vi "LabVIEW_hiss_1.vi"() -> ()   [LabVIEW 2020]
uses:
  States_1.ctl
panel:
  in  "Meta nödstopp":bool
  in  "?":bool
  in  "Tab Control":enum32{"Hisspanel", "Inställningar"}(tab)
  in  "Våningar":T1
  out "Nuvarande Våning":T2
  out "Våningshöjd":dbl
  out "Våningstolerans":dbl
  in  "Potentiometervärden":T3={"Högsta våning"=10.0, "Lägsta våning"=0.0}
  in  "GPIB-addresser":T4={"Funktionsgenerator"="1", "Multimeter"="3", "Nätaggregat"="2"}
  in  "Antal våningar":i32=5
  in  "Tolerans Rel. Våningshöjd":i32=5
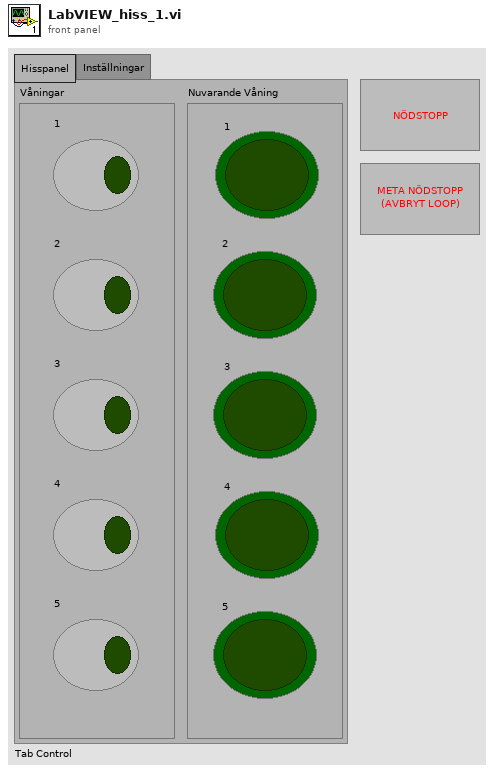
[diagram p1: front panel]
types:
  T1 = cluster{"1":bool, "2":bool, "3":bool, "4":bool, "5":bool}
  T2 = cluster{"1":bool, "\n2":bool, "3":bool, "4":bool, "5":bool}
  T3 = cluster{"Högsta våning":dbl, "Lägsta våning":dbl}
  T4 = cluster{"Funktionsgenerator":string, "Multimeter":string, "Nätaggregat":string}
  T5 = cluster{"Våningshöjd":dbl, "Våningstolerans":dbl, "Högsta våning":dbl, "Lägsta våning":dbl}
  T6 = typedef "States_1.ctl" = enum16{"Initialtillstånd", "Kör ner", "Kör upp", "Vänta på input", "Spela ljudfil", "Nödstopp"}
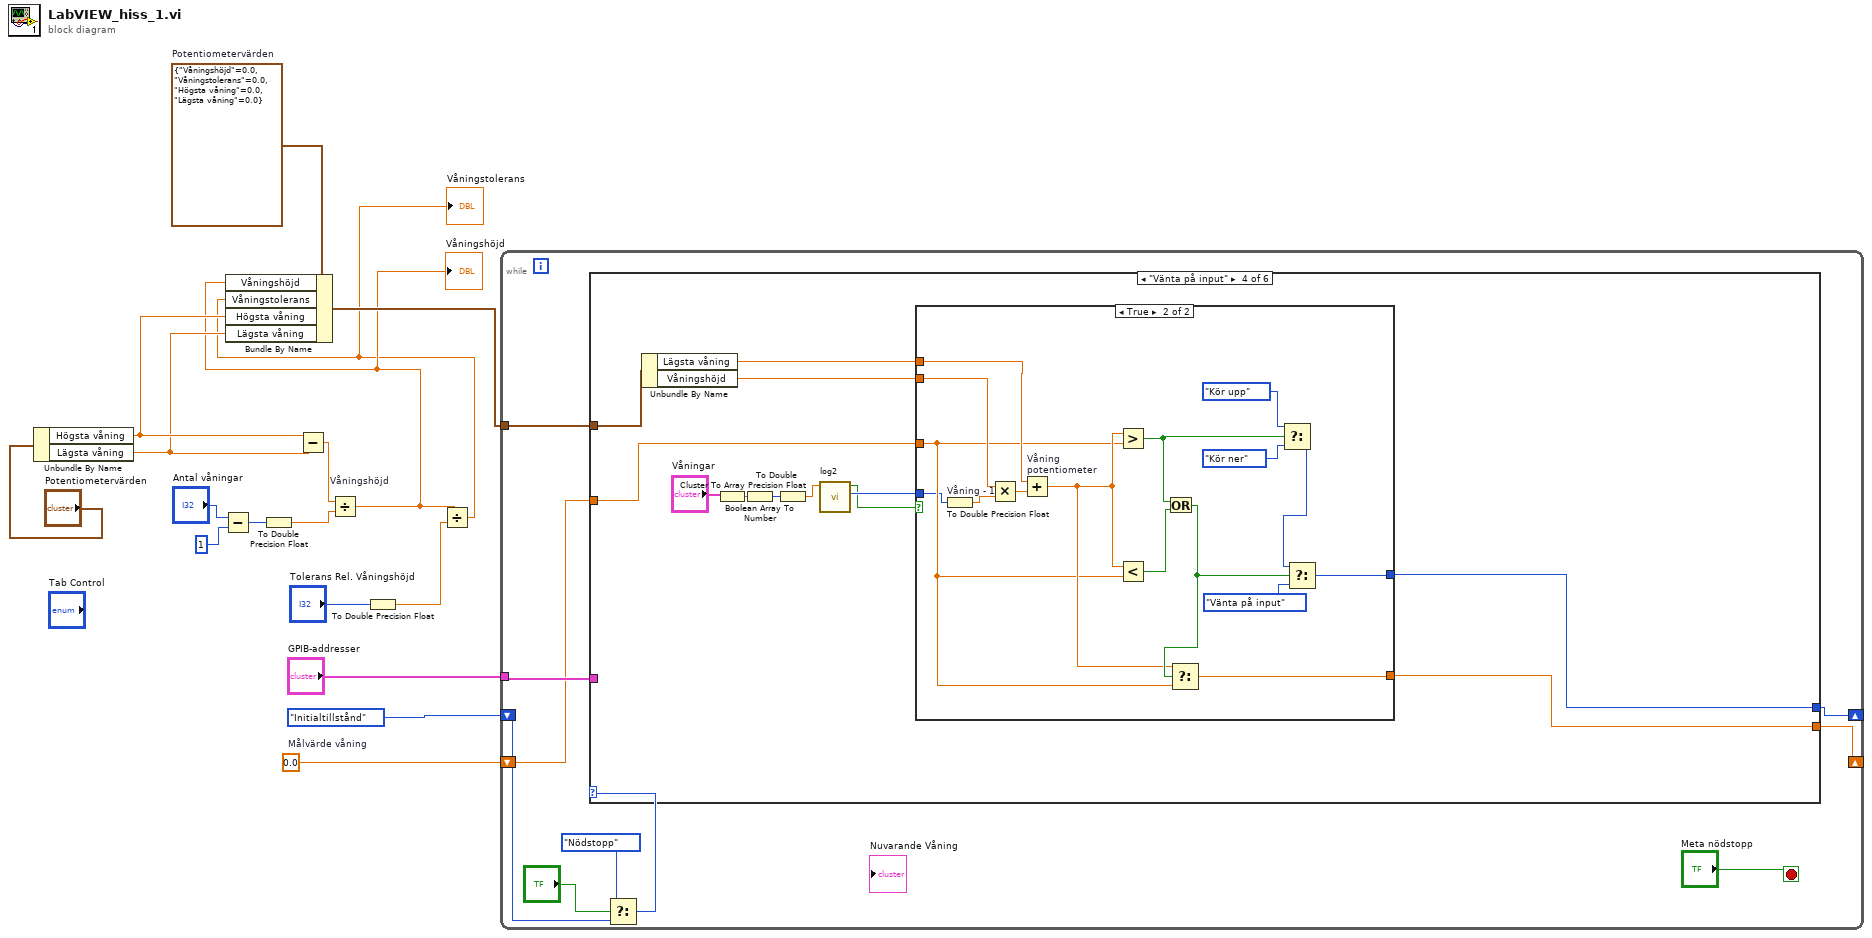
[diagram p0: block diagram]
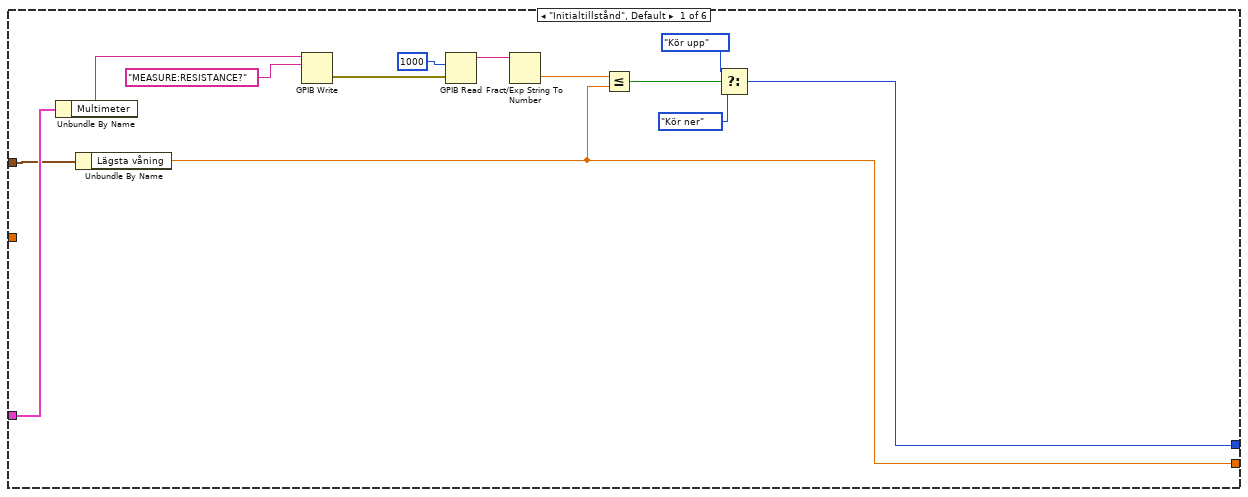
[diagram p2: hidden frame]
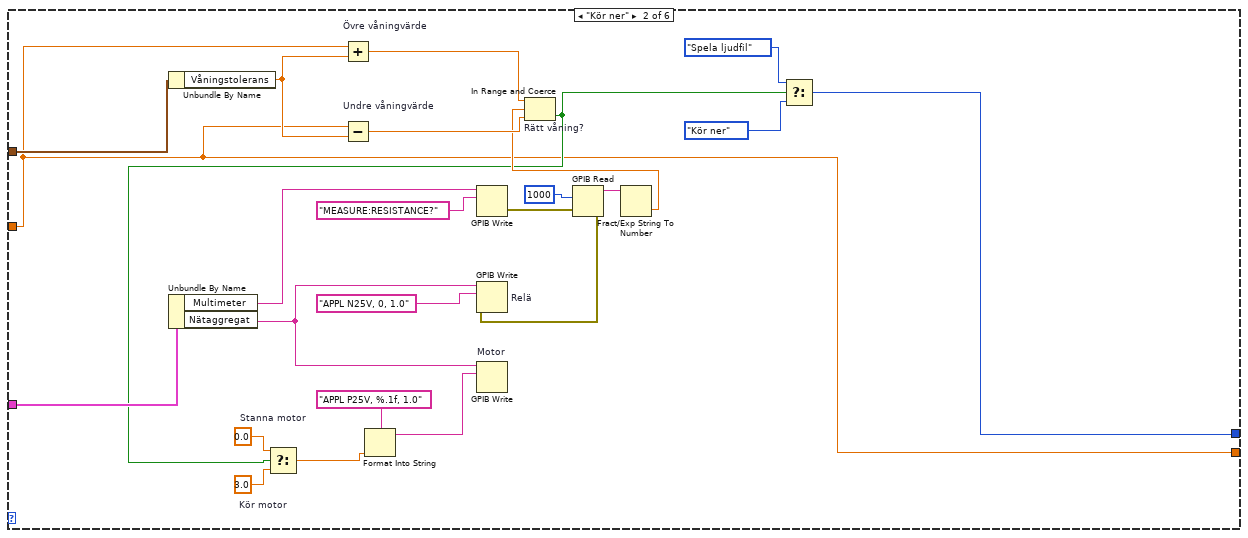
[diagram p3: hidden frame]
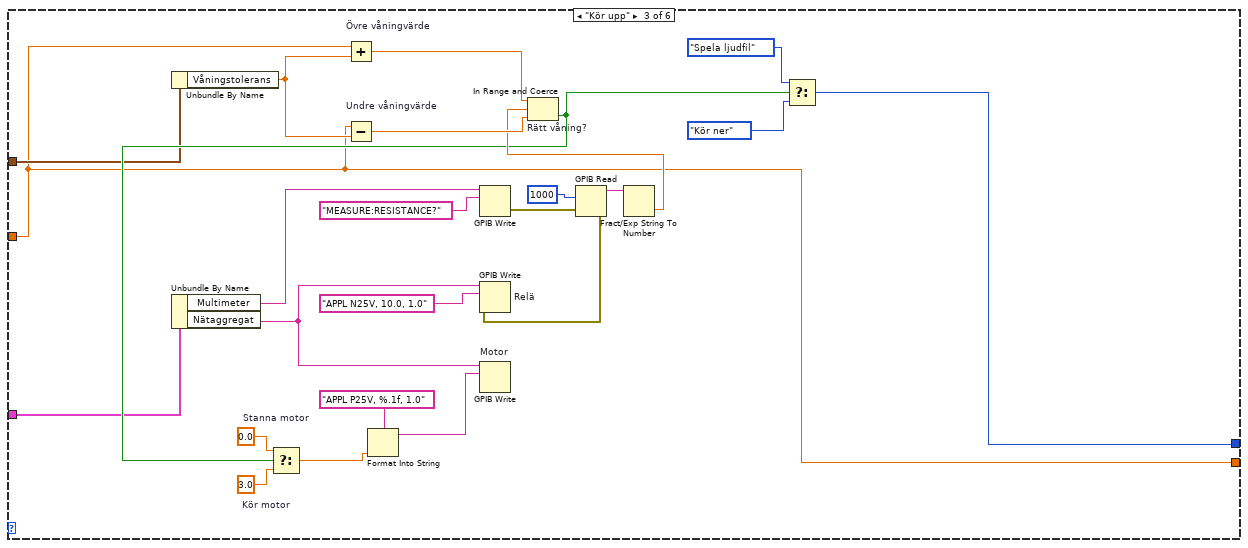
[diagram p4: hidden frame]
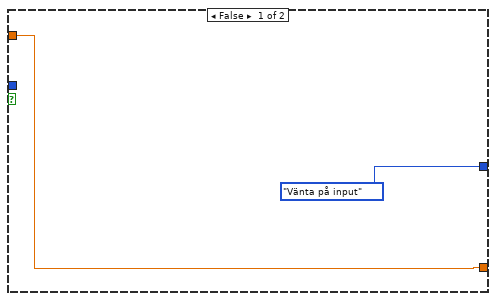
[diagram p5: hidden frame]
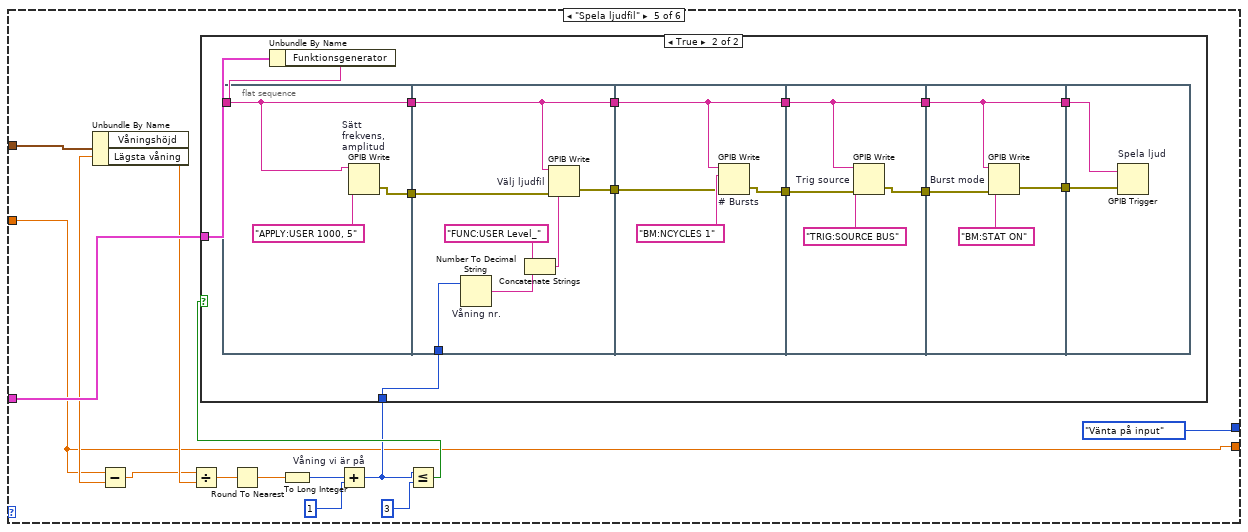
[diagram p6: hidden frame]
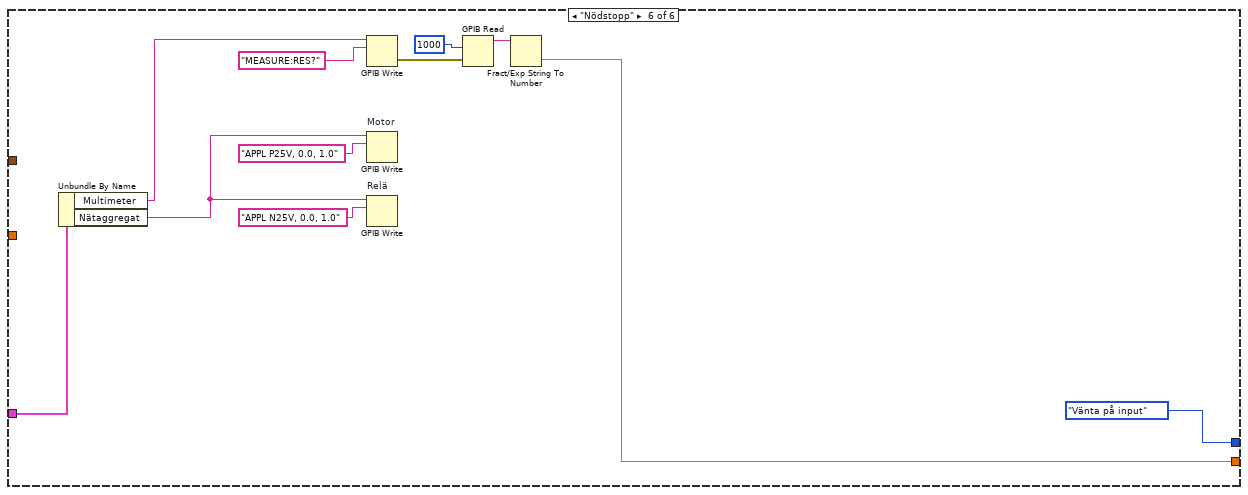
[diagram p8: hidden frame]
diagram:
  w16 = 0.0  # Målvärde våning
  w10 = T5 {"Våningshöjd"=0.0, "Våningstolerans"=0.0, "Högsta våning"=0.0, "Lägsta våning"=0.0}  # Potentiometervärden
  n1 = Unbundle By Name("Potentiometervärden") -> ("Högsta våning"=w5:dbl, "Lägsta våning"=w4:dbl)
  n2 = Subtract(x="Antal våningar", y=1) -> (x-y=w13:i32)
  n3 = To Double Precision Float(number=w13) -> (double precision float=w12:dbl)
  n4 = Subtract(x=w5, y=w4) -> (x-y=w14:dbl)
  n5 = Divide "Våningshöjd"(x=w14, y=w12) -> (x/y=w3:dbl)
  "Våningshöjd" <- w3
  n6 = To Double Precision Float(number="Tolerans Rel. Våningshöjd") -> (double precision float=w11:dbl)
  n7 = Divide(x=w3, y=w11) -> (x/y=w2:dbl)
  "Våningstolerans" <- w2
  n8 = Bundle By Name(cluster=w10, "Våningshöjd"=w3, "Våningstolerans"=w2, "Högsta våning"=w5, "Lägsta våning"=w4) -> (w9:T5)
  n9 = while {
    shift-right: [w22] -> _
    shift-left: States_1."Initialtillstånd" -> [w26]
    tunnel: "GPIB-addresser" -> [w23]
    shift-right: [w21] -> _
    shift-left: w16 -> [w19]
    tunnel: w9 -> [w20]
    stop <- "Meta nödstopp" stop-if-true
    n10 = Select(t=States_1."Nödstopp", s="?", f=w26) -> (s? t:f=w24:T6)
    n11 = case shown="\"Vänta på input\"" w24 {
      tunnel: w23 -> [w40 w63 w66 _ w130 w178]
      tunnel: [w30 w43 w65 w92 States_1."Vänta på input" States_1."Vänta på input"] -> w22
      tunnel: [w29 w41 w64 w90 w117 w170] -> w21
      tunnel: w20 -> [w28 w58 w67 w95 w129 _]
      tunnel: w19 -> [_ w41 w64 w91 w117 _]
      frame "Initialtillstånd", Default {
        n12 = Unbundle By Name(w40) -> ("Multimeter"=w39:string)
        n13 = Unbundle By Name(w28) -> ("Lägsta våning"=w29:dbl)
        n14 = GPIB Write(0:w39, 1:"MEASURE:RESISTANCE?") -> (6:w37:errorcluster)  [unwired: 3 in, 1 out]
        n15 = GPIB Read(1:1000, 3:w37) -> (5:w35:string)  [unwired: 3 in, 2 out]
        n16 = Fract/Exp String To Number(string=w35) -> (number=w34:dbl)  [unwired: 3 in, 1 out]
        n17 = Less Or Equal?(x=w34, y=w29) -> (x <= y?=w33:bool)
        n18 = Select(t=States_1."Kör upp", s=w33, f=States_1."Kör ner") -> (s? t:f=w30:T6)
      }
      frame "Kör ner" {
        w50 = 3.0  # Kör motor
        w51 = 0.0  # Stanna motor
        n19 = Unbundle By Name(w58) -> ("Våningstolerans"=w57:dbl)
        n20 = Unbundle By Name(w63) -> ("Nätaggregat"=w48:string)  [unwired: 1 out]
        n21 = Add "Övre våningvärde"(x=w41, y=w57) -> (x+y=w56:dbl)
        n22 = Subtract "Undre våningvärde"(x=w41, y=w57) -> (x-y=w55:dbl)
        n23 = GPIB Write(0:w48, 1:"MEASURE:RESISTANCE?") -> (6:w61:errorcluster)  [unwired: 3 in, 1 out]
        n24 = GPIB Read(1:1000, 3:w61) -> (5:w59:string, 7:w46:errorcluster)  [unwired: 3 in, 1 out]
        n25 = GPIB Write "Relä"(0:w48, 1:"APPL N25V, 0, 1.0", 3:w46) -> ()  [unwired: 2 in, 2 out]
        n26 = Fract/Exp String To Number(string=w59) -> (number=w54:dbl)  [unwired: 3 in, 1 out]
        n27 = In Range and Coerce "Rätt våning?"(upper limit=w56, x=w54, lower limit=w55) -> (In Range?=w42:bool)  [unwired: 1 out]
        n28 = Select(t=w51, s=w42, f=w50) -> (s? t:f=w49:dbl)
        n29 = Format Into String(format string="APPL P25V, %.1f, 1.0", w49) -> (resulting string=w52:string)  [unwired: 2 in, 1 out]
        n30 = GPIB Write "Motor"(0:w48, 1:w52) -> ()  [unwired: 3 in, 2 out]
        n31 = Select(t=States_1."Spela ljudfil", s=w42, f=States_1."Kör ner") -> (s? t:f=w43:T6)
      }
      frame "Kör upp" {
        w75 = 3.0  # Kör motor
        w76 = 0.0  # Stanna motor
        n32 = Unbundle By Name(w67) -> ("Våningstolerans"=w82:dbl)
        n33 = Unbundle By Name(w66) -> ("Nätaggregat"=w73:string)  [unwired: 1 out]
        n34 = Add "Övre våningvärde"(x=w64, y=w82) -> (x+y=w81:dbl)
        n35 = Subtract "Undre våningvärde"(x=w64, y=w82) -> (x-y=w80:dbl)
        n36 = GPIB Write(0:w73, 1:"MEASURE:RESISTANCE?") -> (6:w85:errorcluster)  [unwired: 3 in, 1 out]
        n37 = GPIB Read(1:1000, 3:w85) -> (5:w83:string, 7:w71:errorcluster)  [unwired: 3 in, 1 out]
        n38 = GPIB Write "Relä"(0:w73, 1:"APPL N25V, 10.0, 1.0", 3:w71) -> ()  [unwired: 2 in, 2 out]
        n39 = Fract/Exp String To Number(string=w83) -> (number=w79:dbl)  [unwired: 3 in, 1 out]
        n40 = In Range and Coerce "Rätt våning?"(upper limit=w81, x=w79, lower limit=w80) -> (In Range?=w68:bool)  [unwired: 1 out]
        n41 = Select(t=w76, s=w68, f=w75) -> (s? t:f=w74:dbl)
        n42 = Format Into String(format string="APPL P25V, %.1f, 1.0", w74) -> (resulting string=w77:string)  [unwired: 2 in, 1 out]
        n43 = GPIB Write "Motor"(0:w73, 1:w77) -> ()  [unwired: 3 in, 2 out]
        n44 = Select(t=States_1."Spela ljudfil", s=w68, f=States_1."Kör ner") -> (s? t:f=w65:T6)
      }
      frame "Vänta på input" {
        n45 = Unbundle By Name(w95) -> ("Lägsta våning"=w93:dbl, "Våningshöjd"=w94:dbl)
        n46 = Cluster To Array(cluster="Våningar") -> (array=w97:bool[])
        n47 = Boolean Array To Number(Boolean array=w97) -> (number=w96:u32)
        n48 = To Double Precision Float(number=w96) -> (double precision float=w89:dbl)
        n49 = call "log2.vi"("Input"=w89) -> ("Numeric"=w88:i32, "Boolean"=w87:bool)  [unwired: 9 in]
        n50 = case shown="True" w87 {
          tunnel: w94 -> [_ w116]
          tunnel: w93 -> [_ w114]
          tunnel: [States_1."Vänta på input" w107] -> w92
          tunnel: w91 -> [w100 w103]
          tunnel: [w100 w104] -> w90
          tunnel: w88 -> [_ w101]
          frame False {
          }
          frame True {
            n51 = To Double Precision Float "Våning - 1"(number=w101) -> (double precision float=w102:dbl)
            n52 = Multiply(x=w116, y=w102) -> (x*y=w115:dbl)
            n53 = Add "Våning\npotentiometer"(x=w114, y=w115) -> (x+y=w105:dbl)
            n54 = Greater?(x=w105, y=w103) -> (0:w112:bool)
            n55 = Less?(x=w105, y=w103) -> (x < y?=w113:bool)
            n56 = Or(x=w112, y=w113) -> (x .or. y?=w106:bool)
            n57 = Select(t=w105, s=w106, f=w103) -> (s? t:f=w104:dbl)
            n58 = Select(t=States_1."Kör upp", s=w112, f=States_1."Kör ner") -> (s? t:f=w108:T6)
            n59 = Select(t=w108, s=w106, f=States_1."Vänta på input") -> (s? t:f=w107:T6)
          }
        }
      }
      frame "Spela ljudfil" {
        n60 = Unbundle By Name(w129) -> ("Våningshöjd"=w127:dbl, "Lägsta våning"=w128:dbl)
        n61 = Subtract(x=w117, y=w128) -> (x-y=w126:dbl)
        n62 = Divide(x=w126, y=w127) -> (x/y=w125:dbl)
        n63 = Round To Nearest(number=w125) -> (nearest integer value=w124:dbl)
        n64 = To Long Integer(number=w124) -> (32bit integer=w123:i32)
        n65 = Add "Våning vi är på"(x=w123, y=1) -> (x+y=w118:i32)
        n66 = Less Or Equal?(x=w118, y=3) -> (x <= y?=w120:bool)
        n67 = case shown="True" w120 {
          tunnel: w130 -> [_ w143]
          tunnel: w118 -> [_ w131]
          frame False {
          }
          frame True {
            n68 = flat-sequence {
              tunnel: w142 -> [w145]
              tunnel: [w145] -> w141
              tunnel: [w144] -> w137
              tunnel: w141 -> [w149]
              tunnel: w131 -> [w153]
              tunnel: [w149] -> w140
              tunnel: w137 -> [w148]
              tunnel: [w147] -> w136
              tunnel: w140 -> [w157]
              tunnel: [w157] -> w139
              tunnel: w136 -> [w155]
              tunnel: [w154] -> w135
              tunnel: w139 -> [w161]
              tunnel: [w161] -> w138
              tunnel: w135 -> [w159]
              tunnel: [w158] -> w134
              tunnel: w138 -> [w165]
              tunnel: w134 -> [w163]
              tunnel: [w165] -> w133
              tunnel: [w162] -> w132
              tunnel: w133 -> [w167]
              tunnel: w132 -> [w166]
              frame #0 {
                n69 = GPIB Write "Sätt\nfrekvens,\namplitud"(0:w145, 1:"APPLY:USER 1000, 5") -> (6:w144:errorcluster)  [unwired: 3 in, 1 out]
              }
              frame #1 {
                n70 = Number To Decimal String "Våning nr."(number=w153) -> (decimal integer string=w151:string)  [unwired: 1 in]
                n71 = Concatenate Strings("FUNC:USER Level_", w151) -> (w150:string)
                n72 = GPIB Write "Välj ljudfil"(0:w149, 1:w150, 3:w148) -> (6:w147:errorcluster)  [unwired: 2 in, 1 out]
              }
              frame #2 {
                n73 = GPIB Write "# Bursts"(0:w157, 1:"BM:NCYCLES 1", 3:w155) -> (6:w154:errorcluster)  [unwired: 2 in, 1 out]
              }
              frame #3 {
                n74 = GPIB Write "Trig source"(0:w161, 1:"TRIG:SOURCE BUS", 3:w159) -> (6:w158:errorcluster)  [unwired: 2 in, 1 out]
              }
              frame #4 {
                n75 = GPIB Write "Burst mode"(0:w165, 1:"BM:STAT ON", 3:w163) -> (6:w162:errorcluster)  [unwired: 2 in, 1 out]
              }
              frame #5 {
                n76 = GPIB Trigger "Spela ljud"(2:w166, 3:w167) -> ()  [unwired: 2 out]
              }
            }
            n77 = Unbundle By Name(w143) -> ("Funktionsgenerator"=w142:string)
          }
        }
      }
      frame "Nödstopp" {
        n78 = Unbundle By Name(w178) -> ("Multimeter"=w168:string, "Nätaggregat"=w175:string)
        n79 = GPIB Write(0:w168, 1:"MEASURE:RES?") -> (6:w173:errorcluster)  [unwired: 3 in, 1 out]
        n80 = GPIB Write "Motor"(0:w175, 1:"APPL P25V, 0.0, 1.0") -> ()  [unwired: 3 in, 2 out]
        n81 = GPIB Write "Relä"(0:w175, 1:"APPL N25V, 0.0, 1.0") -> ()  [unwired: 3 in, 2 out]
        n82 = GPIB Read(1:1000, 3:w173) -> (5:w171:string)  [unwired: 3 in, 2 out]
        n83 = Fract/Exp String To Number(string=w171) -> (number=w170:dbl)  [unwired: 3 in, 1 out]
      }
    }
  }
